vi "_Main.vi"   [LabVIEW 2017, in "DashBoardCom.lvlib"]
uses:
  DashBoardCom.lvlib
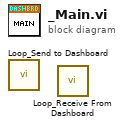
[diagram p0: block diagram]
diagram:
  n1 = call "Loop_Send to Dashboard.vi"() -> ()  [unwired: 12 in]
  n2 = call "Loop_Receive From Dashboard.vi"() -> ()  [unwired: 12 in]
